vi "UnregisterMat_1DArray-3DPoint-SGL.vi"(6 "AdressOrData":T1[](array[typedef]), 8 "error in":errorcluster, 11 "Image":u8) -> (0 "error out":errorcluster, 3 "Datatype":T1[](array[typedef]))   [LabVIEW 2020, in "OpenLvVision_OpenCv.lvlib"]
doc: "Register mat for dll.\nNo malleable to breake vi inlining!"
uses:
  OpenLvVision_OpenCv.lvlib
  TypeDef/Point/3D_PointSGL.ctl
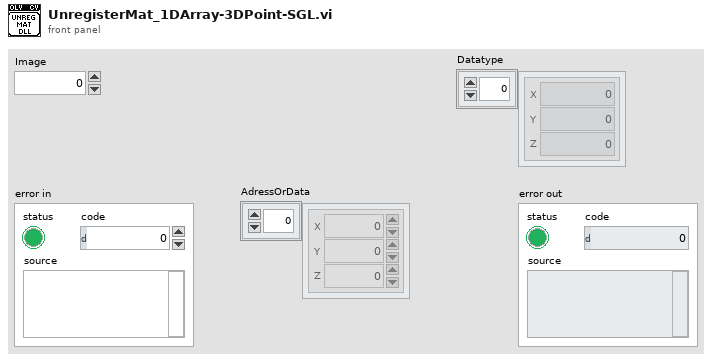
[diagram p1: front panel]
types:
  T1 = typedef "OpenLvVision_OpenCv.lvlib/3D_PointSGL.ctl" = cluster{"X":sgl, "Y":sgl, "Z":sgl}
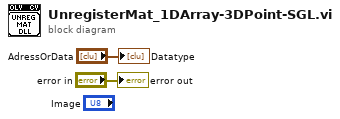
[diagram p0: block diagram]
diagram:
  "error out" <- "error in"
  "Datatype" <- "AdressOrData"
